vi "建立设备.vi"(8 "错误输入":errorcluster caption="错误输入（无错误）") -> (0 "错误输出":errorcluster, 3 "设备句柄":i32=1 min=1 max=50)   [LabVIEW 2016]
uses:
  dll/em9636.dll
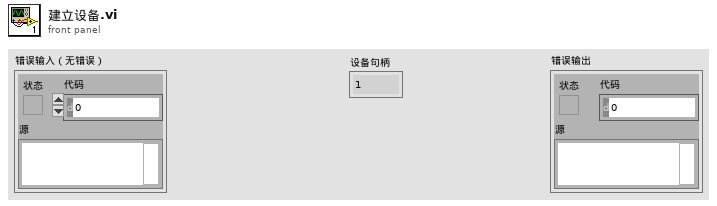
[diagram p1: front panel]
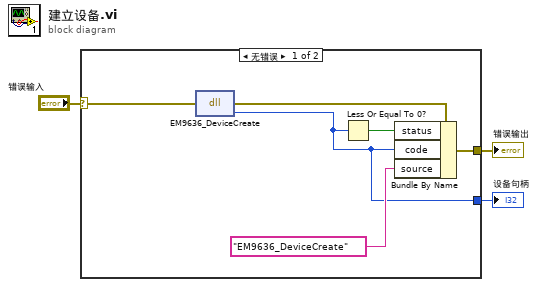
[diagram p0: block diagram]
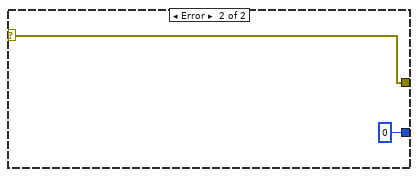
[diagram p2: hidden frame]
diagram:
  n1 = case shown="无错误" "错误输入" {
    selector: "错误输入" -> [w9 w11]
    tunnel: [w5 w11] -> w2
    tunnel: [w4 0 ("错误")] -> w1
    frame No Error {
      n2 = dll-call lib="PTH2kabs CUsers\nAdministratorDesktopEM9636*EM9636系列_demo_labview(调用DLL方式)dll\nem9636.dll" fn="EM9636_DeviceCreate"(error in=w9) -> (error out=w7:errorcluster, "错误"=w4:i32)  [unwired: 2 in, 1 out]
      n3 = Less Or Equal To 0?(x=w4) -> (x <= 0?=w6:bool)
      n4 = Bundle By Name(cluster=w7, "status"=w6, "code"=w4, "source"="EM9636_DeviceCreate") -> (w5:errorcluster)
    }
    frame Error {
    }
  }
  "错误输出" <- w2
  "设备句柄" <- w1
